vi "2_wavelength_subVI.vi"(8 "Input_Intensity":dbl[](array[numeric]), 9 "Input_wavelength":dbl[](array[numeric]), 10 "pixel difference":dbl) -> (0 "Intensity_2":dbl[](array[numeric]), 1 "Intensity_1":dbl[](array[numeric]), 2 "Wavelength_2":dbl[](array[numeric]), 3 "Wavelength_1":dbl[](array[numeric]))   [LabVIEW 2017]
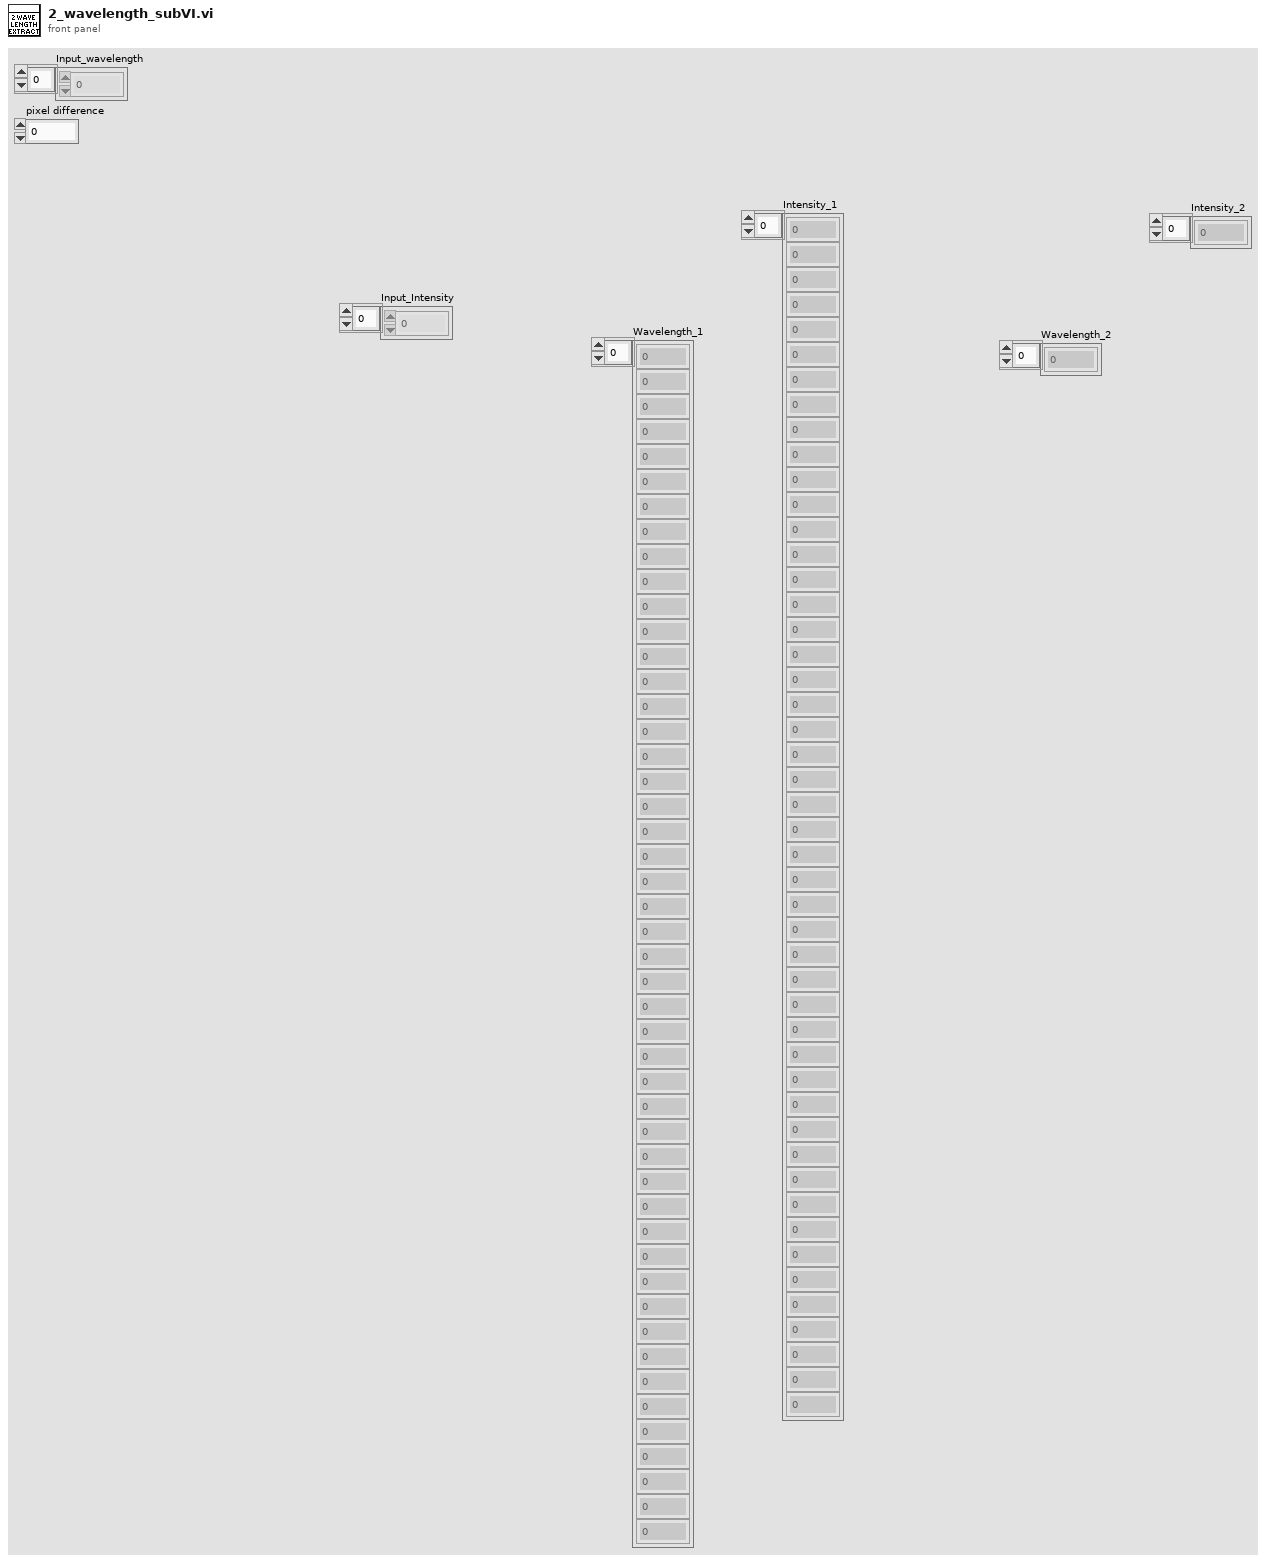
[diagram p1: front panel]
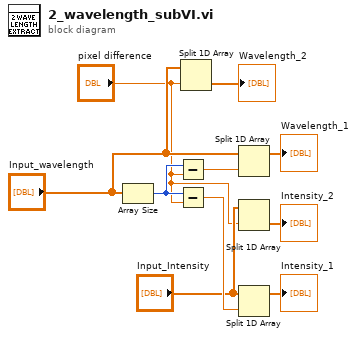
[diagram p0: block diagram]
diagram:
  n1 = Array Size(array="Input_wavelength") -> (size(s)=w2:i32)
  n2 = Subtract(x=w2, y="pixel difference") -> (x-y=w10:dbl)
  n3 = Subtract(x=w2, y="pixel difference") -> (x-y=w7:dbl)
  n4 = Split 1D Array(array="Input_wavelength", index="pixel difference") -> (second subarray=→"Wavelength_2":dbl[])  [unwired: 1 out]
  n5 = Split 1D Array(array="Input_wavelength", index=w10) -> (first subarray=→"Wavelength_1":dbl[])  [unwired: 1 out]
  n6 = Split 1D Array(array="Input_Intensity", index="pixel difference") -> (second subarray=→"Intensity_2":dbl[])  [unwired: 1 out]
  n7 = Split 1D Array(array="Input_Intensity", index=w7) -> (first subarray=→"Intensity_1":dbl[])  [unwired: 1 out]
